vi "Add Fire Pixel Source.vi"(8 "Click Position":cluster{i32, i32}, 9 "Height":i32, 10 "Width":i32, 11 "Pixel Array In":i32[](array[numeric])) -> (3 "Pixel Array Out":i32[](array[numeric]))   [LabVIEW 2019]
doc: "Sets the clicked / dragged pixel position to the fire source, creating a basic particle effect."
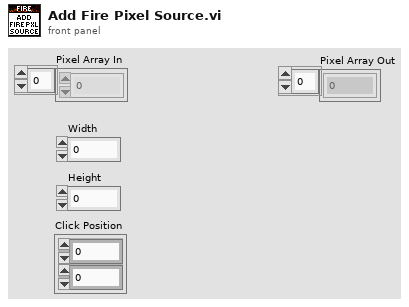
[diagram p1: front panel]
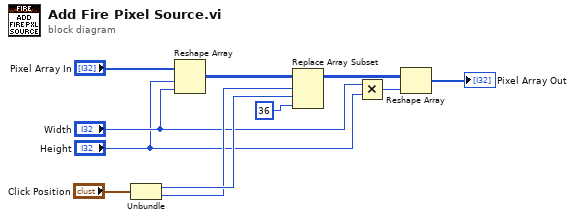
[diagram p0: block diagram]
diagram:
  n1 = Unbundle("Click Position") -> (w8:i32, w7:i32)
  n2 = Reshape Array("Pixel Array In", "Height", "Width") -> (w9:i32[][])
  n3 = Replace Array Subset(array=w9, new element=36 ("f"), index (row)=w7, index (col)=w8) -> (w5:i32[][])
  n4 = Multiply(x="Width", y="Height") -> (x*y=w4:i32)
  n5 = Reshape Array(w5, w4) -> (→"Pixel Array Out":i32[])
